vi "LtaGet.vi"(8 "Error In":errorcluster[](array[cluster]), 10 "arg":string="Doe1.Ray.Mi") -> (0 "Error Out":errorcluster[](array[cluster]))   [LabVIEW 2017, in "Bus_class.lvlib" / "Bus.lvclass"]
uses:
  Bus.lvclass
  Config_class/Config.lvclass/Config.ctl
  Config_class/Accessors/Read PARTF Root Directory.vi
  Config_class/Accessors/Read ConfigFilePath.vi
  Config_class/Read Logging.vi
  <vilib>/Utility/error.llb/Error Cluster From Error Code.vi
  <vilib>/ErrorRing/Error Ring.xnode
  TestAutomation/LTA/LTA.lvlib
  <userlib>/NIST/NISTErrorLib/NISTErrorLib.lvlib
  TestAutomation/Comms/Comms.lvlib
  Framework.lvlib
  Config_class/Config.lvclass
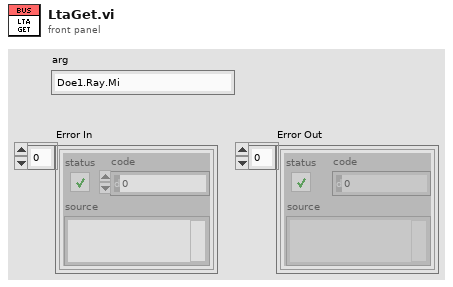
[diagram p1: front panel]
types:
  T1 = typedef "Framework.lvlib/clFrameworkData.ctl" = cluster{"EvtINIFilePaths":path[], "BusClassInstances":refnum<class "Bus.lvclass">[], "PmuImpairINIFilePaths":path[], "FlagImpairINIFilePaths":path[], "NetImpairINIFilePaths":path[], "OutputToFileINIFilePaths":path[], "AppINIFilePaths":path[], "AppModuleID":i32, "OutputToFileID":i32}
  T2 = cluster{"RootDir":path, "TestDir":string, "ScriptDir":string, "OutDir":string, "ConfigFilePath":path, "Log File Path":path}
  T3 = typedef "Framework.lvlib/Config.lvclass/RootDir.ctl" = cluster{"pathRootDir":path, "btnOutPath":bool, "OutDir":string, "btnOpenOutputDir":bool, "ScriptDir":string, "btnOpenScriptDir":bool, "TestDir":string, "btnOpenTestDir":bool}
  T4 = typedef "Framework.lvlib/Config.lvclass/Logging.ctl" = cluster{"eLogLvl":T5, "Log File Path":path, "btnLogFile":bool}
  T5 = typedef "Framework.lvlib/Config.lvclass/eLogLvl.ctl" = enum16{"Normal", "Verbose", "None"}
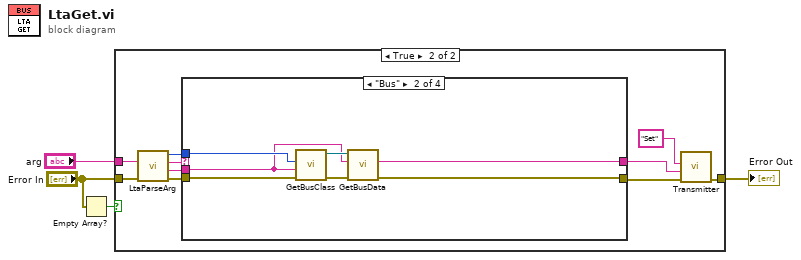
[diagram p0: block diagram]
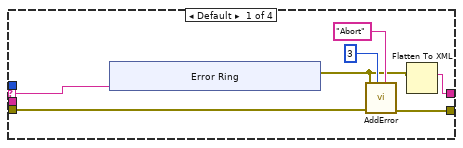
[diagram p3: hidden frame]
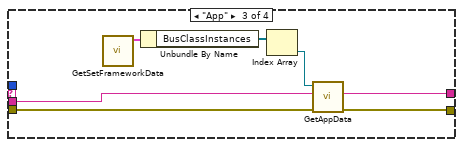
[diagram p4: hidden frame]
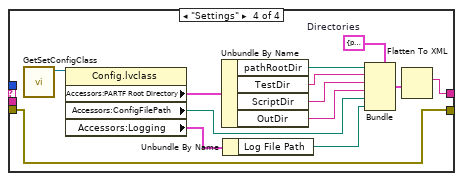
[diagram p5: hidden frame]
diagram:
  n1 = Empty Array?(array="Error In") -> (empty?=w4:bool)
  n2 = case shown="True" w4 {
    tunnel: "Error In" -> [w5 w15]
    tunnel: [w5 w8] -> w2
    tunnel: "arg" -> [_ w14]
    frame False {
    }
    frame True {
      n3 = call "LtaParseArg.vi"("Error In"=w15, "Arg In"=w14) -> ("Error Out"=w10:errorcluster[], "ArgRemaining"=w12:string, "Arg 1"=w13:string, "Arg1Num"=w11:i32)  [unwired: 6 in]
      n4 = case shown="\"Bus\"" w13 {
        selector: w13 -> [w21 _ _ _]
        tunnel: w12 -> [_ w30 w43 _]
        tunnel: w11 -> [_ w35 _ _]
        tunnel: w10 -> [w22 w36 w42 w44]
        tunnel: [w20 w32 w37 w44] -> w9
        tunnel: [w16 w31 w38 w46] -> w7
        frame Default {
          n5 = xnode "Error Ring"("parameter 0"=w21) -> ("error out"=w17:errorcluster)
          n6 = call <userlib>:"AddError.vi"("Severity"="Abort", "Priority"=u8 3, "ErrorArray"=w22, "error in (no error)"=w17) -> ("ErrorArray"=w20:errorcluster[])  [unwired: 6 in, 1 out]
          n7 = Flatten To XML(anything=w17) -> (xml string=w16:string)
        }
        frame "Bus" {
          n8 = call "GetBusClass.vi"("ErrorArray In"=w36, "arg"=w30, "BusNumber"=w35) -> ("ErrorArray Out"=w34:errorcluster[], "Framework.lvlib:Bus.lvclass"=w33:refnum<class "Bus.lvclass">)  [unwired: 7 in]
          n9 = call "GetBusData.vi"("Error In"=w34, "arg"=w30, "Bus in"=w33) -> ("Error Out"=w32:errorcluster[], "XmlData"=w31:string)  [unwired: 6 in, 1 out]
        }
        frame "App" {
          n10 = call "GetSetFrameworkData.vi"() -> ("clFrameworkData Out"=w41:T1)  [unwired: 11 in]
          n11 = Unbundle By Name(w41) -> ("BusClassInstances"=w40:refnum<class "Bus.lvclass">[])
          n12 = Index Array(array=w40) -> (element=w39:refnum<class "Bus.lvclass">)  [unwired: 1 in]
          n13 = call "GetAppData.vi"("Error In"=w42, "arg"=w43, "Bus in"=w39) -> ("Error Out"=w37:errorcluster[], "XmlData"=w38:string)  [unwired: 6 in, 1 out]
        }
        frame "Settings" {
          w56 = T2 {"RootDir"=path "", "TestDir"="", "ScriptDir"="", "OutDir"="", "ConfigFilePath"=path "", "Log File Path"=path ""}  # Directories
          n14 = call "GetSetConfigClass.vi"() -> ("Ref out"=w45:refnum<class "Config.lvclass">)  [unwired: 11 in]
          n15 = property class="Config.lvclass"(reference=w45) -> ("Accessors:PARTF Root Directory"=w47:T3, "Accessors:ConfigFilePath"=w53:path, "Accessors:Logging"=w54:T4)  [unwired: 1 in, 2 out]
          n16 = Unbundle By Name(w47) -> ("pathRootDir"=w48:path, "TestDir"=w49:string, "ScriptDir"=w50:string, "OutDir"=w51:string)
          n17 = Unbundle By Name(w54) -> ("Log File Path"=w55:path)
          n18 = Bundle(cluster=w56, "RootDir"=w48, "TestDir"=w49, "ScriptDir"=w50, "OutDir"=w51, "ConfigFilePath"=w53, "Log File Path"=w55) -> (w52:T2)
          n19 = Flatten To XML(anything=w52) -> (xml string=w46:string)
        }
      }
      n20 = call "Transmitter.vi"("ErrorArray"=w9, "XMLData"=w7, "Command"="Set") -> ("ErrorArray"=w8:errorcluster[])  [unwired: 7 in, 1 out]
    }
  }
  "Error Out" <- w2
